vi "Create Column.vi"(6 "new column units":string, 7 "selected table path":string, 8 "error in (no error)":errorcluster, 9 "new column name":string, 10 "new column data type":string, 11 "Data.PGSQL in":refnum<class "LV-Data.PGSQL.lvclass">) -> (0 "error out":errorcluster, 3 "Data.PGSQL out":refnum<class "LV-Data.PGSQL.lvclass">)   [LabVIEW 2016, in "LV-Data.PGSQL.lvclass"]
uses:
  LV-Data.PGSQL.lvclass
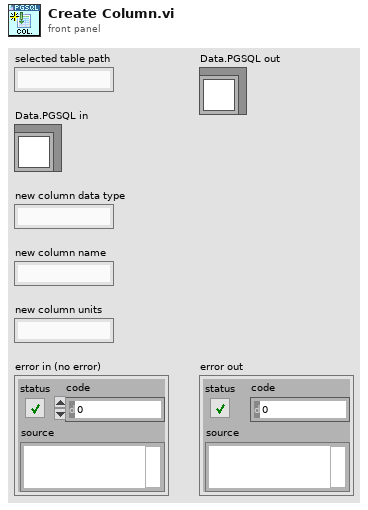
[diagram p1: front panel]
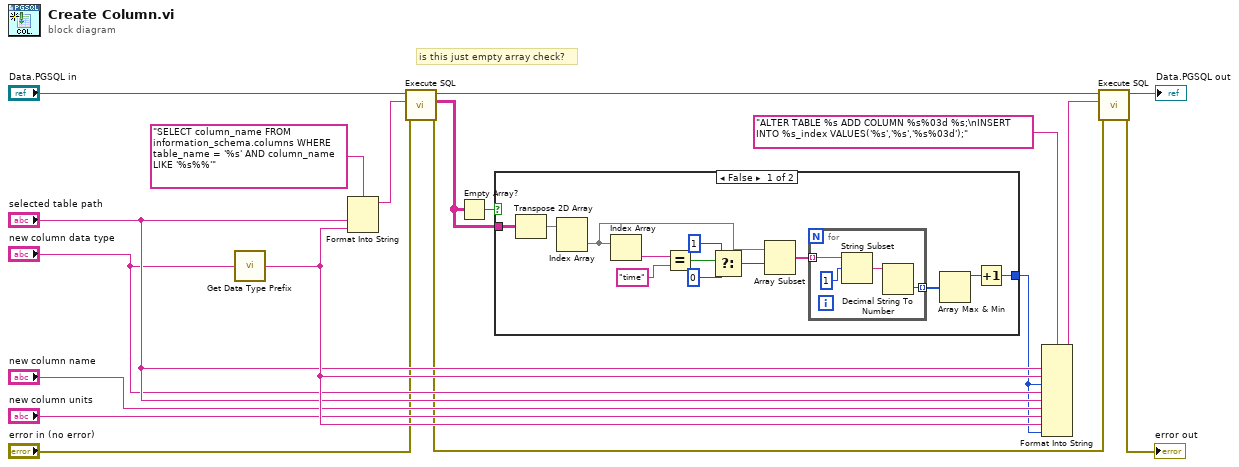
[diagram p0: block diagram]
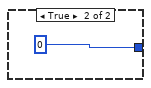
[diagram p2: hidden frame]
diagram:
  # "is this just empty array check?"
  n1 = call "Get Data Type Prefix.vi"("data type in"="new column data type") -> ("data type prefix"=w17:string)
  n2 = Format Into String(format string="SELECT column_name FROM information_schema.columns WHERE table_name = '%s' AND column_name LIKE '%s%%'", "selected table path", w17) -> (resulting string=w5:string)  [unwired: 2 in, 1 out]
  n3 = call "Execute SQL.vi"("error in"="error in (no error)", "SQL"=w5, "Data.PG"="Data.PGSQL in") -> ("error out"=w12:errorcluster, "Result"=w1:string[][], "Data.PG out"=w11:refnum<class "LV-Data.PGSQL.lvclass">)  [unwired: 6 in]
  n4 = Empty Array?(array=w1) -> (empty?=w2:bool)
  n5 = case shown="False" w2 {
    tunnel: w1 -> [w23 _]
    tunnel: [w21 0] -> w6
    frame False {
      n6 = Transpose 2D Array(2D array=w23) -> (transposed array=w31:string[][])
      n7 = Index Array(array=w31) -> (element=w25:string[])  [unwired: 2 in]
      n8 = Index Array(array=w25) -> (element=w30:string)  [unwired: 1 in]
      n9 = Equal?(x=w30, y="time") -> (x = y?=w28:bool)
      n10 = Select(t=1, s=w28, f=0) -> (s? t:f=w27:i32)
      n11 = Array Subset(array=w25, index=w27) -> (w19:string[])  [unwired: 1 in]
      n12 = for {
        tunnel: w19 -> [w35] mode=indexing
        tunnel: [w32] -> w24 mode=indexing
        n13 = String Subset(string=w35, offset (0)=1) -> (substring=w33:string)  [unwired: 1 in]
        n14 = Decimal String To Number(string=w33) -> (number=w32:i32)  [unwired: 2 in, 1 out]
      }
      n15 = Array Max & Min(array=w24) -> (max value=w22:i32)  [unwired: 3 out]
      n16 = Increment(x=w22) -> (x+1=w21:i32)
    }
    frame True {
    }
  }
  n17 = Format Into String(format string="ALTER TABLE %s ADD COLUMN %s%03d %s;\nINSERT INTO %s_index VALUES('%s','%s','%s%03d');", "selected table path", w17, w6, "new column data type", "selected table path", "new column name", "new column units", w17, w6) -> (resulting string=w8:string)  [unwired: 2 in, 1 out]
  n18 = call "Execute SQL.vi"("error in"=w12, "SQL"=w8, "Data.PG"=w11) -> ("error out"=→"error out":errorcluster, "Data.PG out"=→"Data.PGSQL out":refnum<class "LV-Data.PGSQL.lvclass">)  [unwired: 6 in, 1 out]
